vi "Draw_Destinations.vi"(8 "error in (no error)":errorcluster, 9 "defaultDir":string, 10 "Destination":refnum<class "IB_Destination.lvclass">[](array[class]), 11 "IB_DestTree in":refnum<class "IB_Tree_Dest.lvclass">) -> (0 "error out":errorcluster, 3 "IB_DestTree out":refnum<class "IB_Tree_Dest.lvclass">)   [LabVIEW 2020, in "IB_Tree_Dest.lvclass"]
uses:
  <vilib>/AppBuilder/IB_Classes/Tree_Dest/IB_Tree_Dest.lvclass
  <vilib>/AppBuilder/IB_Classes/Tree_Dest/IB_Tree_Dest.lvclass/IB_Tree_Dest.ctl
  <vilib>/AppBuilder/IB_Classes/Tree/IB_Tree.lvclass
  <vilib>/AppBuilder/IB_Classes/Destination/IB_Destination.lvclass
  <resource>/Framework/Providers/Builds/Installer/controls/IB_Tree_DefaultSymbols.ctl
  e:/builds/penguin/labview/branches/2020/dev/dist/vi.lib/AppBuilder/IB_Classes/Tree/IB_Tree.lvclass
  e:/builds/penguin/labview/branches/2020/dev/dist/vi.lib/AppBuilder/IB_Classes/Tree_Dest/IB_Tree_Dest.lvclass
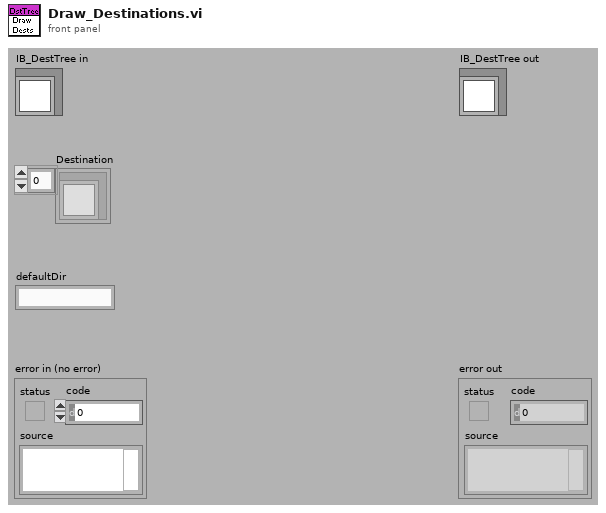
[diagram p1: front panel]
types:
  T1 = typedef "IB_Tree_DefaultSymbols.ctl" = enum16{"<unknown>", "closed folder", "open folder", "closed folder (default)", "open folder (default)", "closed sync folder", "open sync folder", "container folder", "my computer", "build specs", "exe", "dll", "source dist", "restful web service", ".net", "packed library", "c-generator", "target"}
  T2 = typedef "IB_Destination.ctl" = cluster{"name":string, "unlock":bool, "parentTag":string, "destTag":string, "eng_installPath":string}
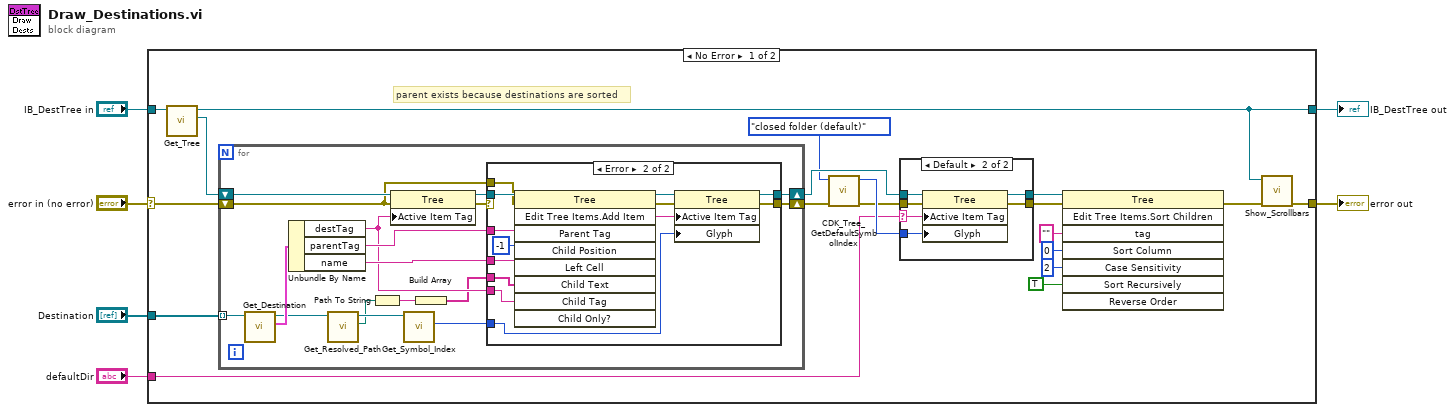
[diagram p0: block diagram]
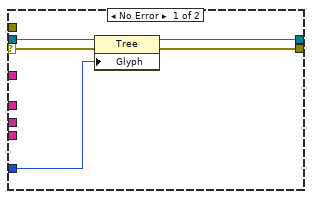
[diagram p3: hidden frame]
diagram:
  n1 = case shown="No Error" "error in (no error)" {
    selector: "error in (no error)" -> [w22 w70]
    tunnel: [w15 w70] -> w5
    tunnel: [w14 w69] -> w3
    tunnel: "IB_DestTree in" -> [w24 w69]
    tunnel: "Destination" -> [w25 _]
    tunnel: "defaultDir" -> [w16 _]
    frame No Error {
      # "parent exists because destinations are sorted"
      n2 = call <vilib>:"Get_Tree.vi"("IB_Tree in"=w24) -> ("ctl"=w23:refnum<vi>, "IB_Tree out"=w14:refnum<class "IB_Tree_Dest.lvclass">)  [unwired: 1 in, 8 out]
      n3 = for {
        tunnel: w25 -> [w50] mode=indexing
        shift-right: [w42] -> w18
        shift-left: w22 -> [w40]
        shift-right: [w39] -> w21
        shift-left: w23 -> [w48]
        n4 = call <vilib>:"Get_Destination.vi"("IB_Destination in"=w50) -> ("data"=w49:T2, "IB_Destination out"=w38:refnum<class "IB_Destination.lvclass">)  [unwired: 1 in, 8 out]
        n5 = Unbundle By Name(w49) -> ("destTag"=w43:string, "parentTag"=w45:string, "name"=w44:string)
        n6 = call-dynamic "Get_Resolved_Path.vi"("IB_Destination in"=w38) -> ("resolved path"=w36:path, "IB_Destination out"=w37:refnum<class "IB_Destination.lvclass">)  [unwired: 8 in, 1 out]
        n7 = Path To String(path=w36) -> (string=w35:string)
        n8 = property class="Tree"(reference=w48, error in=w40, "Active Item Tag"=w43) -> (reference out=w46:refnum<vi>, error out=w47:errorcluster)
        n9 = call-dynamic "Get_Symbol_Index.vi"("IB_Destination in"=w37) -> ("symbol index"=w41:i32)  [unwired: 1 in, 9 out]
        n10 = Build Array(w35) -> (w34:string[])
        n11 = case shown="Error" w47 {
          selector: w47 -> [w54 _]
          tunnel: w46 -> [w55 w68]
          tunnel: [w53 w62] -> w42
          tunnel: w45 -> [_ w67]
          tunnel: w44 -> [_ w66]
          tunnel: w43 -> [_ w65]
          tunnel: w41 -> [w52 w61]
          tunnel: w40 -> [_ w59]
          tunnel: [w51 w58] -> w39
          tunnel: w34 -> [_ w56]
          frame No Error {
            n12 = property class="Tree"(reference=w55, error in=w54, "Glyph"=w52) -> (reference out=w51:refnum<vi>, error out=w53:errorcluster)
          }
          frame Error {
            n13 = invoke class="Tree" method="Edit Tree Items.Add Item"(reference=w68, error in=w59, "Parent Tag"=w67, "Child Position"=-1, "Left Cell"=w66, "Child Text"=w56, "Child Tag"=w65) -> (reference out=w64:refnum<vi>, error out=w63:errorcluster, "Edit Tree Items:Add Item"=w60:string)  [unwired: 2 in, 6 out]
            n14 = property class="Tree"(reference=w64, error in=w63, "Active Item Tag"=w60, "Glyph"=w61) -> (reference out=w58:refnum<vi>, error out=w62:errorcluster)
          }
        }
      }
      n15 = call <resource>:"CDK_Tree_GetDefaultSymbolIndex.vi"("error in (no error)"=w18, "default symbol"=IB_Tree_DefaultSymbols."closed folder (default)") -> ("error out"=w17:errorcluster, "symbol index"=w19:i32)  [unwired: 8 out]
      n16 = case shown="Default" w16 {
        selector: w16 -> [_ w29]
        tunnel: w21 -> [w26 w33]
        tunnel: w19 -> [_ w32]
        tunnel: [w27 w31] -> w12
        tunnel: w17 -> [w27 w30]
        tunnel: [w26 w28] -> w13
        frame "" {
        }
        frame Default {
          n17 = property class="Tree"(reference=w33, error in=w30, "Active Item Tag"=w29, "Glyph"=w32) -> (reference out=w28:refnum<vi>, error out=w31:errorcluster)
        }
      }
      n18 = invoke class="Tree" method="Edit Tree Items.Sort Children"(reference=w13, error in=w12, "tag"="" ("Tag"), "Sort Column"=0, "Case Sensitivity"=2, "Sort Recursively"=TRUE ("Sort Recursively?")) -> (error out=w11:errorcluster)  [unwired: 2 in, 7 out]
      n19 = call <vilib>:"Show_Scrollbars.vi"("error in (no error)"=w11, "IB_Tree in"=w14) -> ("error out"=w15:errorcluster)  [unwired: 9 out]
    }
    frame Error {
    }
  }
  "error out" <- w5
  "IB_DestTree out" <- w3
